vi "STAGE+mono+counter_edit10.vi"() -> ()   [LabVIEW 2017]
uses:
  Control 1.ctl
panel:
  out "Slide":u8(slide) max=10 step=10 scale=0.0..10.0
  out "XY Graph":cluster{dbl[], dbl[]}(graph)
  out "Waveform Graph 2":waveform(dbl)(graph) caption="Record 41  of  100"
  in  "?":enum32{"DELAY", "COUNTER", "MONO"}(tab)
  out "Final time [ps]":dbl
  out "Current time [ps]":dbl
  out "Initial time [ps]":dbl
  in  "Set this as t0":bool
  in  "Axis":i32=1
  in  "Motor ON":bool
  in  "Motor OFF":bool
  out "Current Position [mm]":dbl
  out "Final Position [mm]":dbl
  in  "Data Points":i32=100
  out "Current Point":i32
  in  "Step Size [um]":i32=10
  in  "Target [mm]":dbl format="%.3f"
  in  "Move":bool
  out "Initial position [mm]":dbl
  in  "GPIB address":string="23"
  in  "Count Mode":u16(ring) items=["A,B for Preset T", "A-B for Preset T", "A+B for Preset T", "A for Preset B"]
  in  "Trigger mode":u16(ring) items=["10 MHz"=0, "Input 2"=2, "Input T"=3]
  in  "Channel A Input":u16(ring)=1 items=["10 MHz", "Input 1"]
  in  "Channel B Input":u16(ring)=2 items=["Input 1"=1, "Input 2"=2]
  in  "Number of Measurements\n to take at one point/ Number of Periods":u16=1 min=1 max=2000 step=1
  in  "Time between measurements\n at one point (s)/Dwell Time":dbl=0.002 min=0.002 max=60.0 step=0.001
  in  "gate A mode (CW:0)":i16(slide) scale=0.0..2.0 scale format="%.2f"
  out "Counts":i32
  in  "Integrating time, 10^-7 sec":dbl=10000000.0
  out "Mono port":T1(ring)
  out "Time delay":u32=450000 min=1
  out "Serial":u32=12345
  in  "Step size":dbl=10.0 min=0.0
  in  "Scan to":i32=4000
  in  "Scan from":i32=2600
  out "Current wavelength":dbl
  out "Grt#":u8=1 min=1 max=3 step=1
  in  "?":bool
  out "Groove/mm":u32=1200
  out "Blaze (nm)":u32=300
  out "Timeout 2":bool
  in  "?":bool
  out "Timeout":bool
  in  "Collect Data!":bool
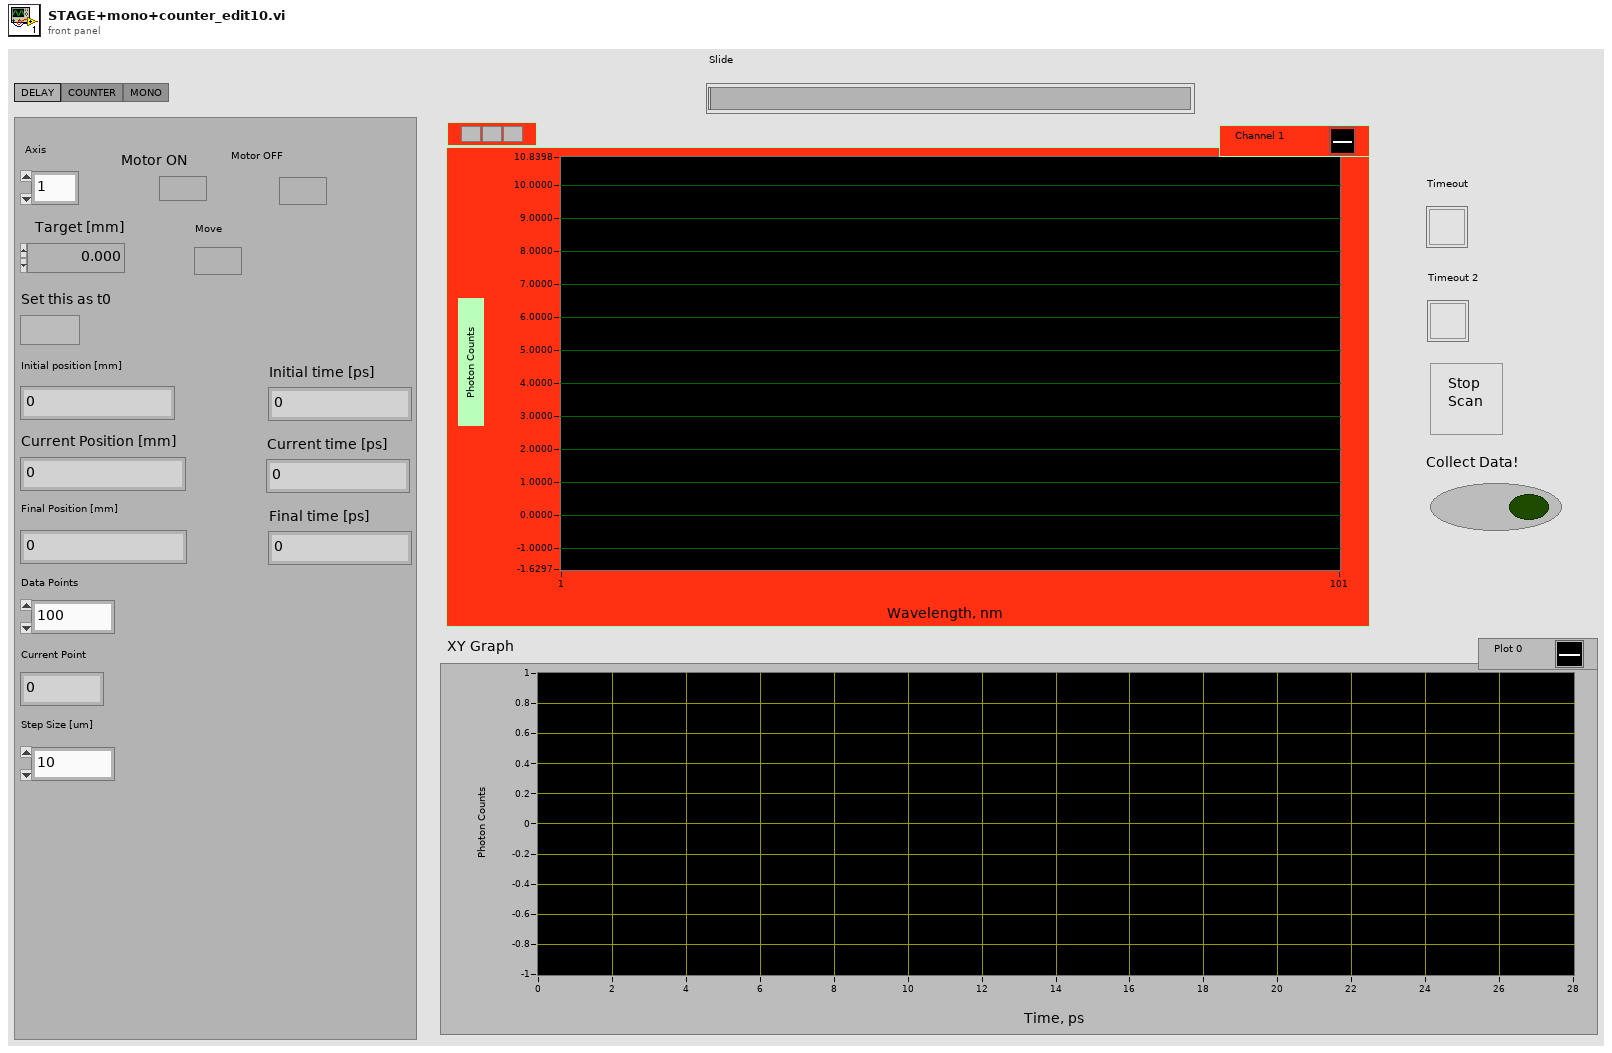
[diagram p1: front panel]
types:
  T1 = enum8{"COM 1", "COM 2", "COM 3", "COM 4", "COM 5", "COM 6", "COM 7", "COM 8", "COM 9"}
  T2 = cluster{"input XON/XOFF":bool, "input HW Handshake":bool, "input alt HW HShk":bool, "output XON/XOFF":bool, "output HW Handshake":bool, "output alt HW HShk":bool, "XOFF byte":u8, "XON byte":u8, "parity error byte":u16}
  T3 = enum16{"no parity", "odd parity", "even parity", "mark parity", "space parity"}
  T4 = typedef "Control 1.ctl" = dbl[]
  T5 = cluster{"Y[0]":dbl, "Y[1]":dbl, "Y[2]":dbl, "Y[3]":dbl, "Y[4]":dbl, "Y[5]":dbl, "Y[6]":dbl, "Y[7]":dbl, "Y[8]":dbl}
  T6 = typedef "NI_Matrix.lvlib/RealMatrix.ctl" = dbl[][]
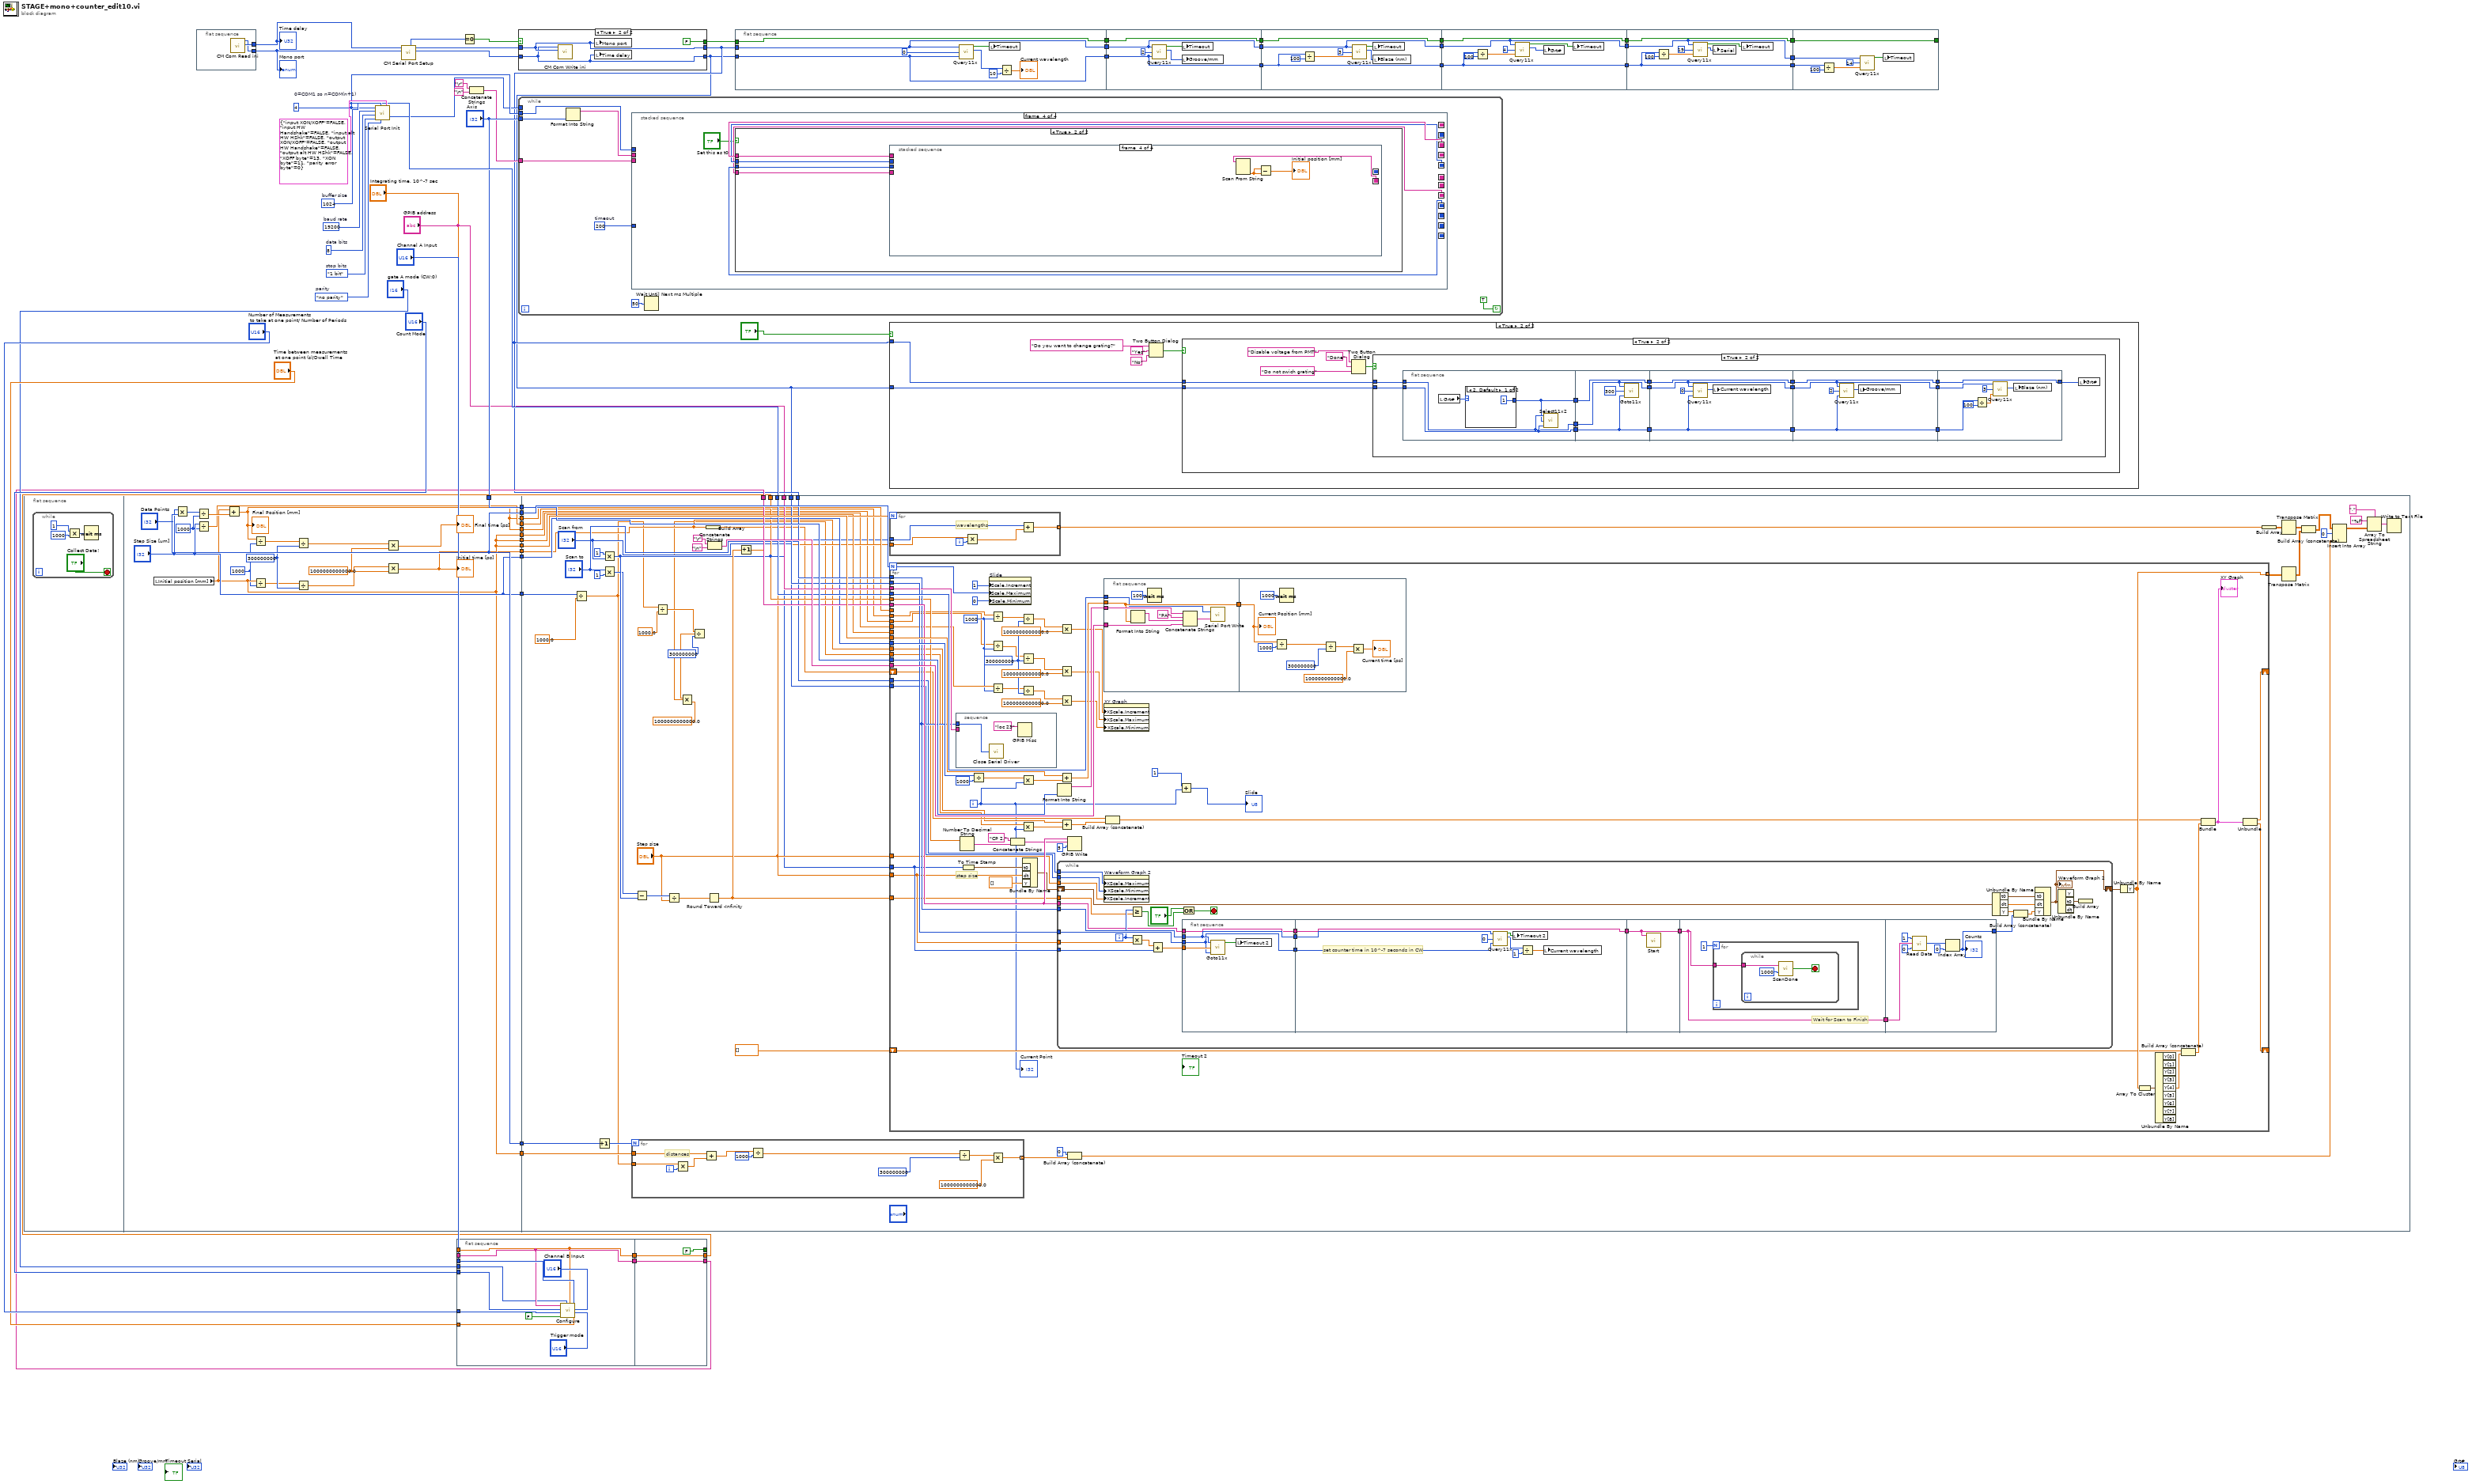
[diagram p0: block diagram]
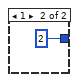
[diagram p5: hidden frame]
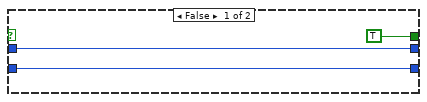
[diagram p6: hidden frame]
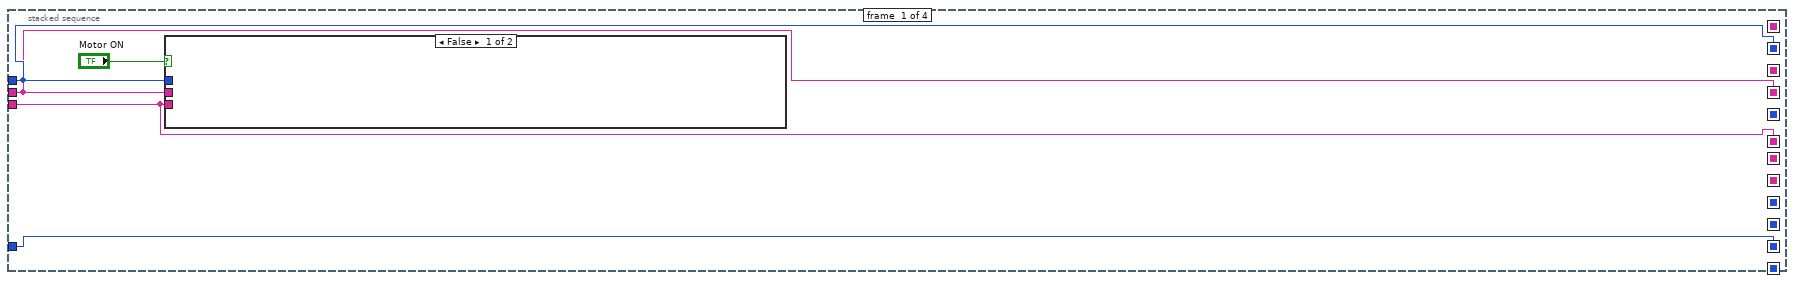
[diagram p7: hidden frame]
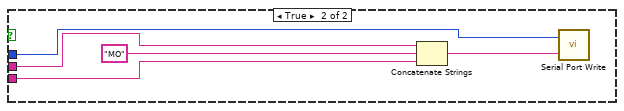
[diagram p8: hidden frame]
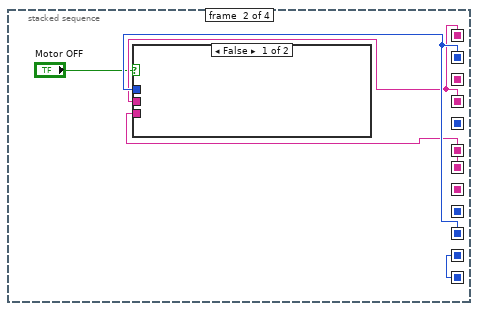
[diagram p9: hidden frame]
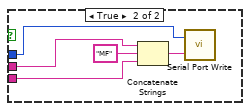
[diagram p10: hidden frame]
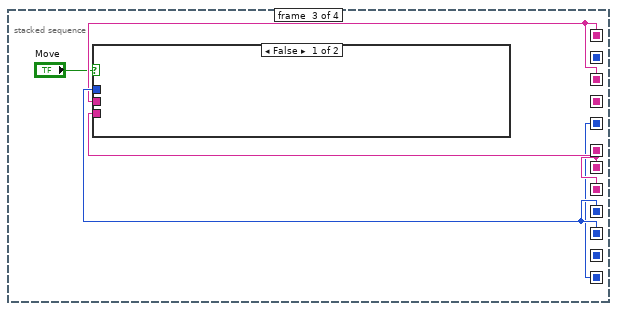
[diagram p11: hidden frame]
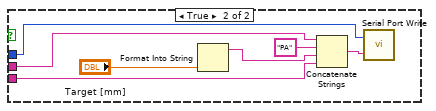
[diagram p12: hidden frame]
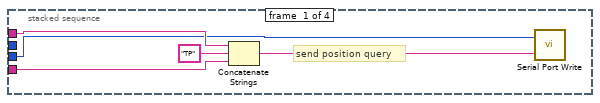
[diagram p14: hidden frame]
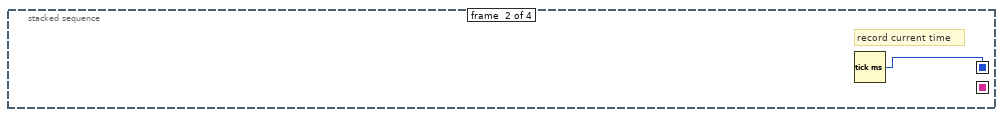
[diagram p15: hidden frame]
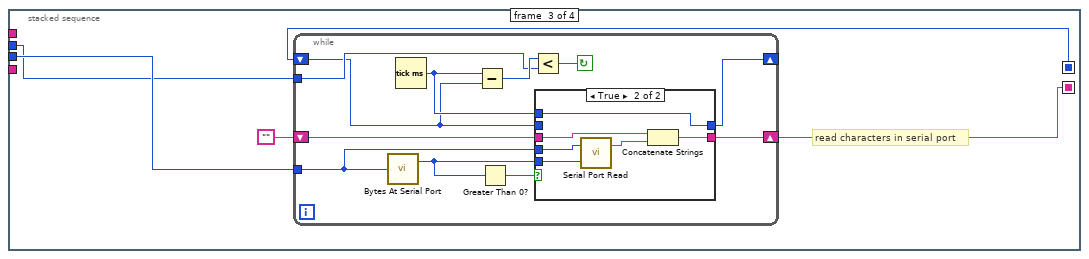
[diagram p16: hidden frame]
diagram:
  w55 = u32 19200  # baud rate
  w54 = u16 8  # data bits
  w53 = enum16{"1 bit", "1.5 bits", "2 bits"}."1 bit"  # stop bits
  w57 = T3."no parity"  # parity
  w52 = 4  # 0=COM1 so n=COM(n+1)
  w56 = u16 1024  # buffer size
  n1 = flat-sequence {
    tunnel: ["Data Points"] -> w61
    tunnel: "Axis" -> [w83]
    tunnel: [w75] -> w60
    tunnel: [w83] -> w59
    tunnel: ["Step Size [um]"] -> w12
    tunnel: [w75] -> w11
    tunnel: ["Step Size [um]"] -> w10
    tunnel: ["Data Points"] -> w9
    tunnel: [w75] -> w8
    tunnel: [w74] -> w7
    tunnel: [w75] -> w4
    tunnel: [w74] -> w3
    tunnel: [w77] -> w2
    tunnel: [w66] -> w1
    tunnel: w61 -> [w141]
    tunnel: w60 -> [w140]
    tunnel: w59 -> [w139]
    tunnel: w52 -> [w135]
    tunnel: w16 -> [w134]
    tunnel: w15 -> [w133]
    tunnel: w14 -> [w132]
    tunnel: "GPIB address" -> [w131]
    tunnel: w12 -> [w116]
    tunnel: w11 -> [w114]
    tunnel: w10 -> [w113]
    tunnel: w9 -> [w111]
    tunnel: w8 -> [w104]
    tunnel: w7 -> [w103]
    tunnel: w6 -> [w102]
    tunnel: w4 -> [w98]
    tunnel: w3 -> [w97]
    tunnel: w2 -> [w96]
    tunnel: w1 -> [w91]
    frame #0 {
      n2 = while {
        stop <- "Collect Data!" stop-if-true
        n3 = Multiply(x=1, y=1000) -> (x*y=w65:i32)
        n4 = Wait (ms)(milliseconds to wait=w65) -> ()  [unwired: 1 out]
      }
    }
    frame #1 {
      w67 = 1000000000000.0
      w73 = 1000
      w76 = 300000000
      w78 = 1000
      n5 = local read "Initial position [mm]"() -> (w75:dbl)
      n6 = Multiply(x="Step Size [um]", y="Data Points") -> (x*y=w82:i32)
      n7 = Divide(x=w82, y=w78) -> (x/y=w81:dbl)
      n8 = Divide(x="Step Size [um]", y=w78) -> (x/y=w77:dbl)
      n9 = Add(x=w75, y=w81) -> (x+y=w74:dbl)
      "Final Position [mm]" <- w74
      n10 = Divide(x=w74, y=w73) -> (x/y=w72:dbl)
      n11 = Divide(x=w75, y=w73) -> (x/y=w71:dbl)
      n12 = Divide(x=w72, y=w76) -> (x/y=w69:dbl)
      n13 = Divide(x=w71, y=w76) -> (x/y=w70:dbl)
      n14 = Multiply(x=w69, y=w67) -> (x*y=→"Final time [ps]":dbl)
      n15 = Multiply(x=w70, y=w67) -> (x*y=w66:dbl)
      "Initial time [ps]" <- w66
    }
    frame #2 {
      n16 = Divide(x=w116, y=1000.0) -> (x/y=w85:dbl)
      n17 = Increment(x=w111) -> (x+1=w112:i32)
      n18 = Multiply(x=1, y="Scan from") -> (x*y=w93:i32)
      n19 = Multiply(x="Scan to", y=1) -> (x*y=w92:i32)
      n20 = for {
        N: w112 -> [_]
        tunnel: w85 -> [w152]
        tunnel: w114 -> [w150]
        tunnel: [w143] -> w110 mode=indexing
        i -> [w151]
        # "distances"
        n21 = Multiply(x=w152, y=w151) -> (x*y=w149:dbl)
        n22 = Add(x=w150, y=w149) -> (x+y=w148:dbl)
        n23 = Divide(x=w148, y=1000) -> (x/y=w142:dbl)
        n24 = Divide(x=w142, y=300000000) -> (x/y=w145:dbl)
        n25 = Multiply(x=w145, y=1000000000000.0) -> (x*y=w143:dbl)
      }
      n26 = Subtract(x=w92, y=w93) -> (x-y=w126:i32)
      n27 = Divide(x=w85, y=1000.0) -> (x/y=w86:dbl)
      n28 = Divide(x=w126, y="Step size") -> (x/y=w125:dbl)
      n29 = Divide(x=w86, y=300000000) -> (x/y=w88:dbl)
      n30 = Multiply(x=w88, y=1000000000000.0) -> (x*y=w84:dbl)
      n31 = Build Array(w91) -> (w94:dbl[])
      n32 = Round Toward -Infinity(1:w125) -> (0:w124:dbl)
      n33 = Concatenate Strings("\r", "\n") -> (w136:string)
      n34 = Increment(x=w124) -> (x+1=w123:dbl)
      n35 = for {
        N: w123 -> [_]
        tunnel: "Step size" -> [w157]
        tunnel: w93 -> [w155]
        tunnel: [w153] -> w121 mode=indexing
        i -> [w156]
        # "wavelengths"
        n36 = Multiply(x=w157, y=w156) -> (x*y=w154:dbl)
        n37 = Add(x=w155, y=w154) -> (x+y=w153:dbl)
      }
      n38 = for {
        N: w141 -> [w181]
        tunnel: w140 -> [w224]
        tunnel: w113 -> [w220]
        tunnel: w139 -> [w217]
        tunnel: w136 -> [w214]
        tunnel: w135 -> [w215]
        tunnel: w134 -> [w213]
        tunnel: w133 -> [w210]
        tunnel: w132 -> [w212]
        tunnel: w131 -> [w211]
        tunnel: [w198] -> w119 mode=indexing
        tunnel: w93 -> [w201]
        tunnel: "Step size" -> [w200]
        tunnel: w124 -> [w199]
        tunnel: w104 -> [_]
        tunnel: w103 -> [_]
        tunnel: w102 -> [w196]
        tunnel: "Scan to" -> [w195]
        tunnel: "Scan from" -> [w194]
        tunnel: "Step size" -> [w193]
        tunnel: w98 -> [w176]
        tunnel: w97 -> [w174]
        tunnel: w96 -> [w177]
        tunnel: w84 -> [w161]
        shift-right: [w191] -> _
        shift-left: w94 -> [w186]
        shift-right: [w188] -> _
        shift-left: T4 [] ("Y") -> [w187]
        tunnel: w91 -> [w185]
        i -> [w160]
        w175 = 1000
        w178 = 300000000
        # "step size"
        n39 = stacked-sequence {
          tunnel: w210 -> [w281]
          tunnel: w211 -> [_]
          frame #0 {
            n40 = call <vilib>:"Close Serial Driver.vi"("port number"=w281) -> ()  [unwired: 1 out]
            n41 = GPIB Misc(0:"loc 23" ("command string")) -> ()  [unwired: 1 in, 3 out]
          }
        }
        n42 = Number To Decimal String(number=w196) -> (decimal integer string=w205:string)  [unwired: 1 in]
        n43 = To Time Stamp(1:w201) -> (0:w208:timestamp)
        n44 = Divide(x=w220, y=1000) -> (x/y=w219:dbl)
        n45 = property on="Slide" class="Slide (strict)"("Scale.Increment"=1, "Scale.Maximum"=w181, "Scale.Minimum"=0) -> ()  [unwired: 2 in, 2 out]
        n46 = Divide(x=w177, y=w175) -> (x/y=w173:dbl)
        n47 = Divide(x=w174, y=w175) -> (x/y=w171:dbl)
        n48 = Divide(x=w176, y=w175) -> (x/y=w172:dbl)
        n49 = Concatenate Strings("CP 2,", w205) -> (w203:string)
        n50 = Divide(x=w173, y=w178) -> (x/y=w167:dbl)
        n51 = Divide(x=w171, y=w178) -> (x/y=w163:dbl)
        n52 = Divide(x=w172, y=w178) -> (x/y=w165:dbl)
        n53 = Multiply(x=w219, y=w160) -> (x*y=w223:dbl)
        n54 = Multiply(x=w161, y=w160) -> (x*y=w192:dbl)
        n55 = Bundle By Name("t0"=w208, "dt"=w200, "Y"=dbl[] []) -> (w207:waveform(dbl))  [unwired: 1 in]
        n56 = Format Into String(w217) -> (resulting string=w216:string)  [unwired: 3 in, 1 out]
        n57 = while {
          tunnel: w210 -> [w252]
          tunnel: w212 -> [w251]
          shift-right: [w226] -> w202
          shift-left: w207 -> [w249]
          tunnel: w213 -> [w241]
          tunnel: w201 -> [w232]
          tunnel: w200 -> [w231]
          tunnel: w199 -> [w230]
          tunnel: w195 -> [w229]
          tunnel: w194 -> [w228]
          tunnel: w193 -> [w227]
          i -> [w246]
          stop <- w250 stop-if-true
          n58 = property on="Waveform Graph 2" class="WFGraph (strict)"("XScale.Maximum"=w229, "XScale.Minimum"=w228, "XScale.Increment"=w227) -> ()  [unwired: 2 in, 2 out]
          n59 = Greater Or Equal?(x=w246, y=w230) -> (x >= y?=w242:bool)
          n60 = Multiply(x=w246, y=w231) -> (x*y=w253:dbl)
          n61 = Add(x=w253, y=w232) -> (x+y=w233:dbl)
          n62 = Or(x="?", y=w242) -> (x .or. y?=w250:bool)
          n63 = flat-sequence {
            tunnel: w233 -> [w258]
            tunnel: w252 -> [w257]
            tunnel: [w257] -> w239
            tunnel: w251 -> [w256]
            tunnel: [w256] -> w238
            tunnel: w241 -> [w254]
            tunnel: [w254] -> w237
            tunnel: w239 -> [w265]
            tunnel: w238 -> [w264]
            tunnel: w237 -> [w262]
            tunnel: [w262] -> w236
            tunnel: w236 -> [w267]
            tunnel: [w267] -> w235
            tunnel: w235 -> [w268]
            tunnel: [w268] -> w234
            tunnel: w234 -> [w275]
            tunnel: [w274] -> w240
            frame #0 {
              n64 = call "Goto11x.vi"("time delay"=w256, "WAVELENGTH"=w258, "port number"=w257) -> ("timeout"=w255:bool)  [unwired: 2 out]
              n65 = local write "Timeout 2"(w255) -> ()
            }
            frame #1 {
              # "set counter time in 10^-7 seconds in CW"
              n66 = call "Query11x.vi"("port number"=w265, "QUERY"=0, "time delay"=w264) -> ("timeout"=w263:bool, "STATUS MESSAGE"=w261:u16)  [unwired: 2 out]
              n67 = local write "Timeout 2"(w263) -> ()
              n68 = Divide(x=w261, y=1) -> (x/y=w260:dbl)
              n69 = local write "Current wavelength"(w260) -> ()
            }
            frame #2 {
              n70 = call "Start.vi"("GPIB Address"=w267) -> ()  [unwired: 9 in]
            }
            frame #3 {
              # "Wait for Scan to Finish"
              n71 = for {
                N: 1 -> [_]
                tunnel: w268 -> [w270]
                n72 = while {
                  tunnel: w270 -> [w271]
                  stop <- w273 stop-if-true
                  n73 = call "ScanDone.vi"("Wait (ms)"=1000, "GPIB Address"=w271) -> ("Scan Finished?"=w273:bool)
                }
              }
            }
            frame #4 {
              n74 = call "Read Data.vi"("Channel Number"=0, "GPIB Address"=w275, "Number of Datapoints"=1) -> ("Data"=w276:i32[])
              n75 = Index Array(array=w276, index=0) -> (element=w274:i32)
              "Counts" <- w274
            }
          }
          n76 = Unbundle By Name(w249) -> ("t0"=w247:timestamp, "dt"=w248:dbl, "Y"=w245:dbl[])
          n77 = Build Array (concatenate)(w245, w240) -> (w244:dbl[])
          n78 = Bundle By Name("t0"=w247, "dt"=w248, "Y"=w244) -> (w226:waveform(dbl))  [unwired: 1 in]
          "Waveform Graph 2" <- w226
          n79 = Unbundle By Name(w226) -> ("t0"=w225:timestamp)  [unwired: 2 out]
          n80 = Build Array(w225) -> ()  [unwired: 1 out]
        }
        n81 = Multiply(x=w167, y=1000000000000.0) -> (x*y=w166:dbl)
        n82 = Multiply(x=w163, y=1000000000000.0) -> (x*y=w162:dbl)
        n83 = Multiply(x=w165, y=1000000000000.0) -> (x*y=w164:dbl)
        n84 = Add(x=w224, y=w223) -> (x+y=w222:dbl)
        n85 = Add(x=w185, y=w192) -> (x+y=w184:dbl)
        n86 = GPIB Write(0:w213, 1:w203, 2:i16 5 ("mode (0)")) -> ()  [unwired: 2 in, 2 out]
        n87 = flat-sequence {
          tunnel: w222 -> [w284]
          tunnel: [w284] -> w218
          tunnel: w214 -> [w286]
          tunnel: w216 -> [w285]
          tunnel: w215 -> [w282]
          tunnel: w218 -> [w295]
          frame #0 {
            n88 = Format Into String(w284) -> (resulting string=w283:string)  [unwired: 3 in, 1 out]
            n89 = Wait (ms)(milliseconds to wait=u32 100) -> ()  [unwired: 1 out]
            n90 = Concatenate Strings(w285, "PA" ("Substring"), w283, w286) -> (w288:string)
            n91 = call <vilib>:"Serial Port Write.vi"("string to write"=w288, "port number"=w282) -> ()  [unwired: 1 out]
          }
          frame #1 {
            n92 = Divide(x=w295, y=1000) -> (x/y=w293:dbl)
            n93 = Wait (ms)(milliseconds to wait=u32 1000) -> ()  [unwired: 1 out]
            n94 = Divide(x=w293, y=300000000) -> (x/y=w292:dbl)
            n95 = Multiply(x=w292, y=1000000000000.0) -> (x*y=→"Current time [ps]":dbl)
            "Current Position [mm]" <- w295
          }
        }
        n96 = property on="XY Graph" class="XYGraph (strict)"("XScale.Increment"=w166, "XScale.Maximum"=w162, "XScale.Minimum"=w164) -> ()  [unwired: 2 in, 2 out]
        n97 = Build Array (concatenate)(w186, w184) -> (w183:dbl[])
        n98 = Add(x=1, y=w160) -> (x+y=→"Slide":i32)
        n99 = Unbundle By Name(w202) -> ("Y"=w198:dbl[])
        n100 = Array To Cluster(array=w198) -> (cluster=w197:T5)
        n101 = Unbundle By Name(w197) -> ("Y[4]"=w190:dbl)  [unwired: 8 out]
        n102 = Build Array (concatenate)(w187, w190) -> (w189:T4)
        n103 = Bundle(w183, "Y"=w189) -> (w182:cluster{dbl[], "Y":T4})  [unwired: 1 in]
        "XY Graph" <- w182
        n104 = Unbundle(w182) -> (w191:dbl[], "Y"=w188:T4)
        "Current Point" <- w160
      }
      n105 = Build Array (concatenate)(0, w110) -> (w107:dbl[])
      n106 = Build Array(w121) -> (w120:dbl[][])
      n107 = Transpose Matrix(1:w120) -> (0:w118:dbl[][])
      n108 = Transpose Matrix(1:w119) -> (0:w117:dbl[][])
      n109 = Build Array (concatenate)(w118, w117) -> (w106:T6)
      n110 = Insert Into Array(array=w106, index (row)=0, new element=w107) -> (w105:T6)  [unwired: 1 in]
      n111 = Array To Spreadsheet String(delimiter (Tab)=",", array=w105, 3:"%f" ("format string")) -> (spreadsheet string=w122:string)
      n112 = Write to Text File(text=w122) -> ()  [unwired: 3 in, 3 out]
    }
  }
  n113 = flat-sequence {
    tunnel: [w299] -> w30
    tunnel: [w298] -> w29
    frame #0 {
      n114 = call "CM Com Read ini.vi"() -> ("Mono port"=w298:T1, "time delay1"=w299:u32)  [unwired: 7 in]
    }
  }
  n115 = call <vilib>:"Serial Port Init.vi"("flow control etc."=T2 {"input XON/XOFF"=FALSE, "input HW Handshake"=FALSE, "input alt HW HShk"=FALSE, "output XON/XOFF"=FALSE, "output HW Handshake"=FALSE, "output alt HW HShk"=FALSE, "XOFF byte"=13, "XON byte"=11, "parity error byte"=0}, "parity"=w57, "buffer size"=w56, "stop bits"=w53, "data bits"=w54, "baud rate"=w55, "port number"=w52) -> ("error code"=w51:i32)
  n116 = call "CM Serial Port Setup.vi"("COM port"=w29, "time delay"=w30) -> ("time delay1"=w25:u32, "DK port Out"=w26:T1, "error code"=w28:i32)  [unwired: 7 in]
  n117 = flat-sequence {
    tunnel: "GPIB address" -> [w307]
    tunnel: [w307] -> w31
    tunnel: "Count Mode" -> [w308]
    tunnel: "Number of Measurements\n to take at one point/ Number of Periods" -> [w305]
    tunnel: "Time between measurements\n at one point (s)/Dwell Time" -> [w304]
    tunnel: "Channel A Input" -> [w309]
    tunnel: "gate A mode (CW:0)" -> [w301]
    tunnel: "Integrating time, 10^-7 sec" -> [w300]
    tunnel: [w300] -> w5
    tunnel: w31 -> [w311]
    tunnel: [w311] -> w16
    tunnel: [FALSE] -> _
    tunnel: [w310] -> w6
    tunnel: w5 -> [w310]
    frame #0 {
      n118 = call "Configure.vi"("Dwell Time (s)"=w304, "Channel T Input"="Trigger mode", "Channel B Input"="Channel B Input", "Channel A Input"=w309, "Integrating time, 10^-7 sec"=w300, "gate mode (CW:0)"=w301, "Scan End Mode"=FALSE, "Number of Periods"=w305, "Count Mode"=w308, "GPIB Address"=w307) -> ()
    }
    frame #1 {
    }
  }
  n119 = Equal To 0?(x=w28) -> (x = 0?=w27:bool)
  n120 = Concatenate Strings("\r", "\n") -> (w47:string)
  n121 = case shown="True" w27 {
    tunnel: w26 -> [w315 w318]
    tunnel: w25 -> [w314 w317]
    tunnel: [w315 w318] -> w15
    tunnel: [w314 w317] -> w14
    tunnel: [TRUE FALSE] -> w24
    frame False {
    }
    frame True {
      n122 = call "CM Com Write ini.vi"("time delay1"=w318, "Mono port"=w317) -> ()  [unwired: 7 in]
      n123 = local write "Mono port"(w318) -> ()
      n124 = local write "Time delay"(w317) -> ()
    }
  }
  n125 = while {
    tunnel: w52 -> [w321]
    tunnel: w47 -> [w322]
    tunnel: w51 -> [_]
    tunnel: "Axis" -> [w319]
    stop <- TRUE continue-if-true
    w320 = u32 200  # timeout
    n126 = Format Into String(w319) -> (resulting string=w323:string)  [unwired: 3 in, 1 out]
    n127 = stacked-sequence {
      seq-local: [w328 _ _ _] -> [_ w339 _ _]
      seq-local: [w327 _ _ _] -> [_ w338 _ _]
      seq-local: [w329 _ _ _] -> [_ w340 _ _]
      seq-local: [w326 _ _ _] -> [_ w336 _ _]
      seq-local: [_ w339 _ _] -> [_ _ w349 _]
      seq-local: [_ w338 _ _] -> [_ _ w348 _]
      seq-local: [_ w340 _ _] -> [_ _ w350 _]
      seq-local: [_ w336 _ _] -> [_ _ w346 _]
      seq-local: [_ _ w349 _] -> [_ _ _ w362]
      seq-local: [_ _ w348 _] -> [_ _ _ w359]
      seq-local: [_ _ w350 _] -> [_ _ _ w361]
      seq-local: [_ _ w346 _] -> [_ _ _ w360]
      tunnel: w323 -> [w328 _ _ _]
      tunnel: w322 -> [w327 _ _ _]
      tunnel: w321 -> [w329 _ _ _]
      tunnel: w320 -> [w326 _ _ _]
      frame #0 {
        n128 = case shown="False" "Motor ON" {
          tunnel: w329 -> [_ w335]
          tunnel: w328 -> [_ w332]
          tunnel: w327 -> [_ w331]
          frame False {
          }
          frame True {
            n129 = Concatenate Strings(w332, "MO" ("Substring"), w331) -> (w333:string)
            n130 = call <vilib>:"Serial Port Write.vi"("string to write"=w333, "port number"=w335) -> ()  [unwired: 1 out]
          }
        }
      }
      frame #1 {
        n131 = case shown="False" "Motor OFF" {
          tunnel: w340 -> [_ w345]
          tunnel: w339 -> [_ w342]
          tunnel: w338 -> [_ w341]
          frame False {
          }
          frame True {
            n132 = Concatenate Strings(w342, "MF" ("Substring"), w341) -> (w343:string)
            n133 = call <vilib>:"Serial Port Write.vi"("string to write"=w343, "port number"=w345) -> ()  [unwired: 1 out]
          }
        }
      }
      frame #2 {
        n134 = case shown="False" "Move" {
          tunnel: w350 -> [_ w357]
          tunnel: w349 -> [_ w354]
          tunnel: w348 -> [_ w353]
          frame False {
          }
          frame True {
            n135 = Format Into String("Target [mm]") -> (resulting string=w351:string)  [unwired: 3 in, 1 out]
            n136 = Concatenate Strings(w354, "PA" ("Substring"), w351, w353) -> (w355:string)
            n137 = call <vilib>:"Serial Port Write.vi"("string to write"=w355, "port number"=w357) -> ()  [unwired: 1 out]
          }
        }
      }
      frame #3 {
        n138 = case shown="True" "Set this as t0" {
          tunnel: w362 -> [_ w366]
          tunnel: w361 -> [_ w365]
          tunnel: w360 -> [_ w364]
          tunnel: w359 -> [_ w363]
          frame False {
          }
          frame True {
            n139 = stacked-sequence {
              seq-local: [_ w372 _ _] -> [_ _ w374 _]
              seq-local: [_ _ w373 _] -> [_ _ _ w399]
              tunnel: w366 -> [w369 _ _ _]
              tunnel: w365 -> [w368 _ w377 _]
              tunnel: w364 -> [_ _ w375 _]
              tunnel: w363 -> [w367 _ _ _]
              frame #0 {
                # "send position query"
                n140 = Concatenate Strings(w369, "TP" ("Substring"), w367) -> (w370:string)
                n141 = call <vilib>:"Serial Port Write.vi"("string to write"=w370, "port number"=w368) -> ()  [unwired: 1 out]
              }
              frame #1 {
                # "record current time"
                n142 = Tick Count (ms)() -> (millisecond timer value=w372:u32)
              }
              frame #2 {
                # "read characters in serial port"
                n143 = while {
                  shift-left: w374 -> [w378]
                  shift-right: [w379] -> _
                  tunnel: w375 -> [w382]
                  shift-left: "" -> [w385]
                  shift-right: [w384] -> w373
                  tunnel: w377 -> [w386]
                  stop <- w381 continue-if-true
                  n144 = call <vilib>:"Bytes At Serial Port.vi"("port number"=w386) -> ("byte count"=w387:u32)  [unwired: 1 out]
                  n145 = Tick Count (ms)() -> (millisecond timer value=w380:u32)
                  n146 = Subtract(x=w380, y=w378) -> (x-y=w383:u32)
                  n147 = Greater Than 0?(x=w387) -> (x > 0?=w388:bool)
                  n148 = Less?(x=w383, y=w382) -> (x < y?=w381:bool)
                  n149 = case shown="True" w388 {
                    tunnel: w387 -> [_ w396]
                    tunnel: w386 -> [_ w395]
                    tunnel: w385 -> [w390 w393]
                    tunnel: [w390 w392] -> w384
                    tunnel: [w389 w391] -> w379
                    tunnel: w380 -> [_ w391]
                    tunnel: w378 -> [w389 _]
                    frame False {
                    }
                    frame True {
                      n150 = call <vilib>:"Serial Port Read.vi"("requested byte count"=w396, "port number"=w395) -> ("string read"=w394:string)  [unwired: 1 out]
                      n151 = Concatenate Strings(w393, w394) -> (w392:string)
                    }
                  }
                }
              }
              frame #3 {
                n152 = Scan From String(input string=w399) -> (output 1=w397:dbl)  [unwired: 4 in, 3 out]
                n153 = Subtract(x=w397, y=w397) -> (x-y=→"Initial position [mm]":dbl)
              }
            }
          }
        }
      }
    }
    n154 = Wait Until Next ms Multiple(millisecond multiple=u32 50) -> ()  [unwired: 1 out]
  }
  n155 = flat-sequence {
    tunnel: w14 -> [w405]
    tunnel: [w405] -> w46
    tunnel: w15 -> [w407]
    tunnel: [w407] -> w45
    tunnel: w24 -> [w403]
    tunnel: [w403] -> w44
    tunnel: w46 -> [w410]
    tunnel: [w410] -> w43
    tunnel: w45 -> [w412]
    tunnel: [w412] -> w42
    tunnel: w44 -> [w408]
    tunnel: [w408] -> w41
    tunnel: w43 -> [w420]
    tunnel: [w420] -> w40
    tunnel: w42 -> [w417]
    tunnel: [w417] -> w39
    tunnel: w41 -> [w414]
    tunnel: [w414] -> w38
    tunnel: w40 -> [w428]
    tunnel: [w428] -> w37
    tunnel: w39 -> [w425]
    tunnel: [w425] -> w36
    tunnel: w38 -> [w422]
    tunnel: [w422] -> w35
    tunnel: w37 -> [w436]
    tunnel: [w436] -> w34
    tunnel: w36 -> [w433]
    tunnel: [w433] -> w33
    tunnel: w35 -> [w430]
    tunnel: [w430] -> w32
    tunnel: w34 -> [w443]
    tunnel: w33 -> [w440]
    tunnel: [w438] -> _
    tunnel: w32 -> [w438]
    frame #0 {
      n156 = call "Query11x.vi"("port number"=w407, "QUERY"=u16 0, "time delay"=w405) -> ("timeout"=w404:bool, "STATUS MESSAGE"=w402:u16)  [unwired: 2 out]
      n157 = local write "Timeout"(w404) -> ()
      n158 = Divide(x=w402, y=10 ("Numeric")) -> (x/y=→"Current wavelength":dbl)
    }
    frame #1 {
      n159 = call "Query11x.vi"("port number"=w412, "QUERY"=u16 2, "time delay"=w410) -> ("timeout"=w409:bool, "STATUS MESSAGE"=w411:u16)  [unwired: 2 out]
      n160 = local write "Timeout"(w409) -> ()
      n161 = local write "Groove/mm"(w411) -> ()
    }
    frame #2 {
      n162 = Divide(x=w420, y=i16 100 ("device (1)")) -> (x/y=w418:dbl)
      n163 = call "Query11x.vi"("port number"=w417, "QUERY"=u16 3, "time delay"=w418) -> ("timeout"=w415:bool, "STATUS MESSAGE"=w416:u16)  [unwired: 2 out]
      n164 = local write "Timeout"(w415) -> ()
      n165 = local write "Blaze (nm)"(w416) -> ()
    }
    frame #3 {
      n166 = Divide(x=w428, y=i16 100 ("device (1)")) -> (x/y=w426:dbl)
      n167 = call "Query11x.vi"("port number"=w425, "QUERY"=u16 4, "time delay"=w426) -> ("timeout"=w423:bool, "STATUS MESSAGE"=w424:u16)  [unwired: 2 out]
      n168 = local write "Grt#"(w424) -> ()
      n169 = local write "Timeout"(w423) -> ()
    }
    frame #4 {
      n170 = Divide(x=w436, y=i16 100 ("device (1)")) -> (x/y=w434:dbl)
      n171 = call "Query11x.vi"("port number"=w433, "QUERY"=u16 19, "time delay"=w434) -> ("timeout"=w431:bool, "STATUS MESSAGE"=w432:u16)  [unwired: 2 out]
      n172 = local write "Serial"(w432) -> ()
      n173 = local write "Timeout"(w431) -> ()
    }
    frame #5 {
      n174 = Divide(x=w443, y=i16 100 ("device (1)")) -> (x/y=w441:dbl)
      n175 = call "Query11x.vi"("port number"=w440, "QUERY"=u16 14, "time delay"=w441) -> ("timeout"=w439:bool)  [unwired: 3 out]
      n176 = local write "Timeout"(w439) -> ()
    }
  }
  n177 = case shown="True" "?" {
    tunnel: w14 -> [_ w446]
    tunnel: w15 -> [_ w445]
    frame False {
    }
    frame True {
      n178 = Two Button Dialog(message="Do you want to change grating?", 1:"No" ("F button name (\"Cancel\")"), 2:"Yes" ("T button name (\"OK\")")) -> (T button?=w447:bool)
      n179 = case shown="True" w447 {
        tunnel: w446 -> [_ w452]
        tunnel: w445 -> [_ w451]
        frame False {
        }
        frame True {
          n180 = Two Button Dialog(message="Disable voltage from PMT", 1:"Do not swich grating" ("F button name (\"Cancel\")"), 2:"Done" ("T button name (\"OK\")")) -> (T button?=w453:bool)
          n181 = case shown="True" w453 {
            tunnel: w452 -> [_ w471]
            tunnel: w451 -> [_ w470]
            frame False {
            }
            frame True {
              n182 = flat-sequence {
                tunnel: w471 -> [w475]
                tunnel: [w475] -> w468
                tunnel: w470 -> [w474]
                tunnel: [w474] -> w467
                tunnel: [w472] -> w466
                tunnel: w468 -> [w479]
                tunnel: [w479] -> w465
                tunnel: w467 -> [w480]
                tunnel: [w480] -> w464
                tunnel: w466 -> [w478]
                tunnel: [w478] -> w463
                tunnel: w465 -> [w486]
                tunnel: [w486] -> w462
                tunnel: w464 -> [w485]
                tunnel: [w485] -> w461
                tunnel: w463 -> [w483]
                tunnel: [w483] -> w460
                tunnel: w462 -> [w489]
                tunnel: [w489] -> w459
                tunnel: w461 -> [w490]
                tunnel: [w490] -> w458
                tunnel: w460 -> [w487]
                tunnel: [w487] -> w457
                tunnel: w459 -> [w494]
                tunnel: w458 -> [w495]
                tunnel: [w492] -> w469
                tunnel: w457 -> [w492]
                frame #0 {
                  n183 = local read "Grt#"() -> (w473:u8)
                  n184 = case shown="2, Default" w473 {
                    tunnel: [1 2] -> w472
                    frame 2, Default {
                    }
                    frame 1 {
                    }
                  }
                  n185 = call "Select11x2.vi"("time delay"=w475, "NEW GRT?"=w472, "port number"=w474) -> ()  [unwired: 3 out]
                }
                frame #1 {
                  n186 = call "Goto11x.vi"("time delay"=w479, "WAVELENGTH"=u16 300, "port number"=w480) -> ()  [unwired: 3 out]
                }
                frame #2 {
                  n187 = call "Query11x.vi"("port number"=w485, "QUERY"=u16 0, "time delay"=w486) -> ("STATUS MESSAGE"=w482:u16)  [unwired: 3 out]
                  n188 = local write "Current wavelength"(w482) -> ()
                }
                frame #3 {
                  n189 = call "Query11x.vi"("port number"=w490, "QUERY"=u16 2, "time delay"=w489) -> ("STATUS MESSAGE"=w488:u16)  [unwired: 3 out]
                  n190 = local write "Groove/mm"(w488) -> ()
                }
                frame #4 {
                  n191 = Divide(x=w494, y=i16 100 ("device (1)")) -> (x/y=w496:dbl)
                  n192 = call "Query11x.vi"("port number"=w495, "QUERY"=u16 3, "time delay"=w496) -> ("STATUS MESSAGE"=w493:u16)  [unwired: 3 out]
                  n193 = local write "Blaze (nm)"(w493) -> ()
                }
              }
              n194 = local write "Grt#"(w469) -> ()
            }
          }
        }
      }
    }
  }
  "Mono port" <- w29
  "Time delay" <- w30
